vi "SetHiSpeedDeviceGPIOs.vi"(2 "error in (no error)":errorcluster, 3 "Input Output Pins":T1, 4 "Chip Select Pins":T2, 5 "Handle":u32) -> (0 "error out":errorcluster, 1 "Result":u32)   [LabVIEW 2010]
uses:
  FTCSPI.dll
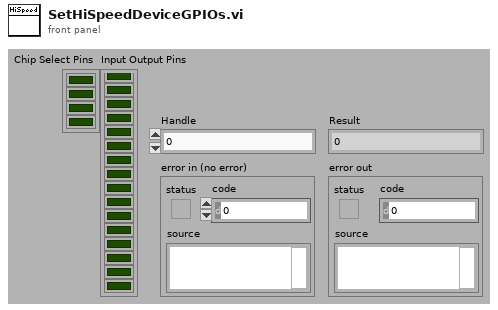
[diagram p1: front panel]
types:
  T1 = cluster{"Boolean":bool, "Boolean 2":bool, "Boolean 3":bool, "Boolean 4":bool, "Boolean 5":bool, "Boolean 6":bool, "Boolean 7":bool, "Boolean 8":bool, "Boolean 9":bool, "Boolean 10":bool, "Boolean 11":bool, "Boolean 12":bool, "Boolean 13":bool, "Boolean 14":bool, "Boolean 15":bool, "Boolean 16":bool}
  T2 = cluster{"Boolean":bool, "Boolean 2":bool, "Boolean 3":bool, "Boolean 4":bool}
  T3 = cluster{u32, u32, u32, u32, u32, u32, u32, u32, u32, u32, u32, u32, u32, u32, u32, u32}
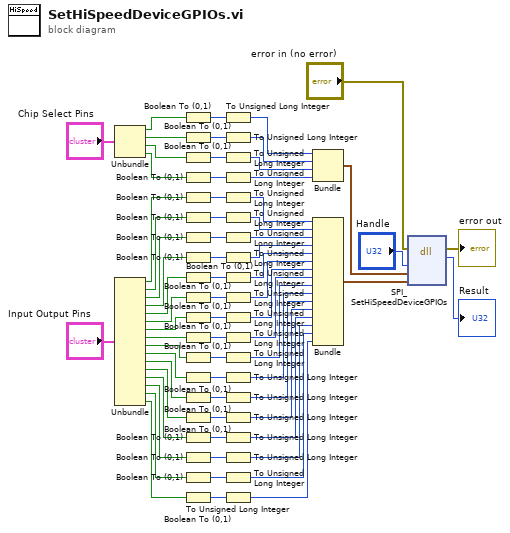
[diagram p0: block diagram]
diagram:
  n1 = Unbundle("Chip Select Pins") -> ("Boolean"=w63:bool, "Boolean 2"=w62:bool, "Boolean 3"=w61:bool, "Boolean 4"=w60:bool)
  n2 = Unbundle("Input Output Pins") -> ("Boolean"=w49:bool, "Boolean 2"=w47:bool, "Boolean 3"=w48:bool, "Boolean 4"=w46:bool, "Boolean 5"=w45:bool, "Boolean 6"=w44:bool, "Boolean 7"=w43:bool, "Boolean 8"=w42:bool, "Boolean 9"=w41:bool, "Boolean 10"=w40:bool, "Boolean 11"=w39:bool, "Boolean 12"=w38:bool, "Boolean 13"=w37:bool, "Boolean 14"=w36:bool, "Boolean 15"=w35:bool, "Boolean 16"=w34:bool)
  n3 = Boolean To (0,1)(Boolean=w63) -> (0, 1=w59:i16)
  n4 = Boolean To (0,1)(Boolean=w62) -> (0, 1=w57:i16)
  n5 = Boolean To (0,1)(Boolean=w61) -> (0, 1=w58:i16)
  n6 = Boolean To (0,1)(Boolean=w60) -> (0, 1=w56:i16)
  n7 = Boolean To (0,1)(Boolean=w49) -> (0, 1=w33:i16)
  n8 = Boolean To (0,1)(Boolean=w47) -> (0, 1=w32:i16)
  n9 = Boolean To (0,1)(Boolean=w48) -> (0, 1=w31:i16)
  n10 = Boolean To (0,1)(Boolean=w46) -> (0, 1=w30:i16)
  n11 = Boolean To (0,1)(Boolean=w45) -> (0, 1=w29:i16)
  n12 = Boolean To (0,1)(Boolean=w44) -> (0, 1=w28:i16)
  n13 = Boolean To (0,1)(Boolean=w43) -> (0, 1=w27:i16)
  n14 = Boolean To (0,1)(Boolean=w42) -> (0, 1=w26:i16)
  n15 = Boolean To (0,1)(Boolean=w41) -> (0, 1=w25:i16)
  n16 = Boolean To (0,1)(Boolean=w40) -> (0, 1=w24:i16)
  n17 = Boolean To (0,1)(Boolean=w39) -> (0, 1=w23:i16)
  n18 = Boolean To (0,1)(Boolean=w38) -> (0, 1=w22:i16)
  n19 = Boolean To (0,1)(Boolean=w37) -> (0, 1=w21:i16)
  n20 = Boolean To (0,1)(Boolean=w36) -> (0, 1=w20:i16)
  n21 = Boolean To (0,1)(Boolean=w35) -> (0, 1=w19:i16)
  n22 = Boolean To (0,1)(Boolean=w34) -> (0, 1=w18:i16)
  n23 = To Unsigned Long Integer(number=w59) -> (unsigned 32bit integer=w55:u32)
  n24 = To Unsigned Long Integer(number=w57) -> (unsigned 32bit integer=w54:u32)
  n25 = To Unsigned Long Integer(number=w58) -> (unsigned 32bit integer=w53:u32)
  n26 = To Unsigned Long Integer(number=w56) -> (unsigned 32bit integer=w52:u32)
  n27 = To Unsigned Long Integer(number=w33) -> (unsigned 32bit integer=w17:u32)
  n28 = To Unsigned Long Integer(number=w32) -> (unsigned 32bit integer=w16:u32)
  n29 = To Unsigned Long Integer(number=w31) -> (unsigned 32bit integer=w15:u32)
  n30 = To Unsigned Long Integer(number=w30) -> (unsigned 32bit integer=w14:u32)
  n31 = To Unsigned Long Integer(number=w29) -> (unsigned 32bit integer=w13:u32)
  n32 = To Unsigned Long Integer(number=w28) -> (unsigned 32bit integer=w12:u32)
  n33 = To Unsigned Long Integer(number=w27) -> (unsigned 32bit integer=w11:u32)
  n34 = To Unsigned Long Integer(number=w26) -> (unsigned 32bit integer=w10:u32)
  n35 = To Unsigned Long Integer(number=w25) -> (unsigned 32bit integer=w9:u32)
  n36 = To Unsigned Long Integer(number=w24) -> (unsigned 32bit integer=w8:u32)
  n37 = To Unsigned Long Integer(number=w23) -> (unsigned 32bit integer=w7:u32)
  n38 = To Unsigned Long Integer(number=w22) -> (unsigned 32bit integer=w6:u32)
  n39 = To Unsigned Long Integer(number=w21) -> (unsigned 32bit integer=w5:u32)
  n40 = To Unsigned Long Integer(number=w20) -> (unsigned 32bit integer=w4:u32)
  n41 = To Unsigned Long Integer(number=w19) -> (unsigned 32bit integer=w3:u32)
  n42 = To Unsigned Long Integer(number=w18) -> (unsigned 32bit integer=w2:u32)
  n43 = Bundle(w55, w54, w53, w52) -> (w51:cluster{u32, u32, u32, u32})  [unwired: 1 in]
  n44 = Bundle(w17, w16, w15, w14, w13, w12, w11, w10, w9, w8, w7, w6, w5, w4, w3, w2) -> (w1:T3)  [unwired: 1 in]
  n45 = dll-call lib="C:/Users/Administrator/Documents/GitHub/labview/FPGA/FTCSPI.dll" fn="SPI_SetHiSpeedDeviceGPIOs"(error in="error in (no error)", "ftHandle"="Handle", "pChipSelectsDisableStates"=w51, "pHighInputOutputPinsData"=w1) -> (error out=→"error out":errorcluster, "result"=→"Result":u32)  [unwired: 5 in, 1 out]
